vi "Configure MX+B.vi"(0 "VISA resource name":refnum<visa-resource-name>, 5 "error in (no error)":errorcluster, 6 "State":bool, 9 "MM Factor":dbl, 11 "MB Factor":dbl) -> (14 "VISA resource name out":refnum<visa-resource-name>, 19 "error out":errorcluster)   [LabVIEW 2020, in "Keithley 2100 Series.lvlib"]
doc: "Definition:\nThis mathematical function multiplies a measurement reading (X) by a specified scale factor (M) and add an offset (B) automatically. The answer (Y) will then be shown on the display according to the following equation.\n\nY=MX+B\n\nThis is especially useful when user needs to do slope calculations on a series of measurements.\nThe values of the “M” and “B” can be changed through the configuration of this function and they are stored in a volatile memory and will be cleared after the meter has been turned off or a remote interface reset.\n\nRemote Interface Operation:\n\nUse the following commands to enable and configure MX+B function:\n\nCALCulate:FUNCtion MXB\nCALCulate:STATe {OFF|ON}\nCALCulate:STATe?\nCALCulate:MXB:MMFactor {<value>|MINimum|MAXimum}\nCALCulate:MXB:MMFactor? [MINimum|MAXimum]\nCALCulate:MXB:MBFactor {<value>|MINimum|MAXimum}\nCALCulate:MXB:MBFactor? [MINimum|MAXimum]"
uses:
  Keithley 2100 Series.lvlib
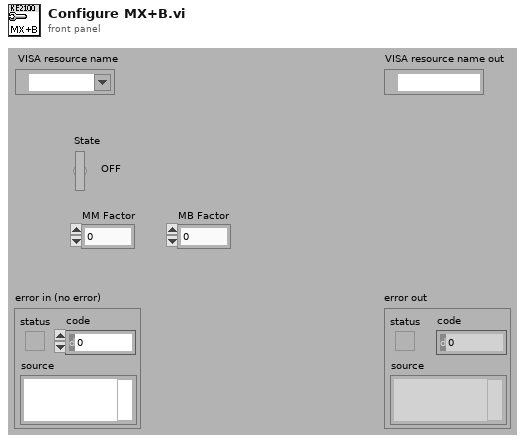
[diagram p1: front panel]
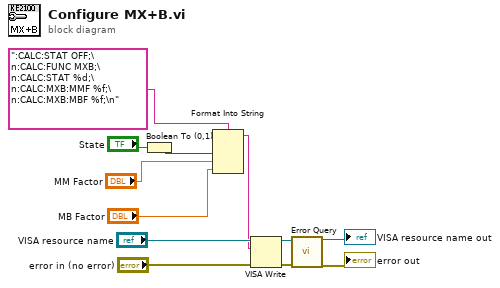
[diagram p0: block diagram]
diagram:
  n1 = Boolean To (0,1)(Boolean="State") -> (0, 1=w5:i16)
  n2 = Format Into String(format string=":CALC:STAT OFF;\n:CALC:FUNC MXB;\n:CALC:STAT %d;\n:CALC:MXB:MMF %f;\n:CALC:MXB:MBF %f;\n", w5, "MM Factor", "MB Factor") -> (resulting string=w6:string)  [unwired: 2 in, 1 out]
  n3 = VISA Write(VISA resource name="VISA resource name", write buffer=w6, error in (no error)="error in (no error)") -> (VISA resource name out=w11:refnum<visa-resource-name>, error out=w12:errorcluster)  [unwired: 1 out]
  n4 = call "Error Query.vi"("VISA resource name"=w11, "error in (no error)"=w12) -> ("VISA resource name out"=→"VISA resource name out":refnum<visa-resource-name>, "error out"=→"error out":errorcluster)  [unwired: 14 in, 2 out]
